vi "Circus FPGA List.vi"(6 "Init":bool, 8 "error in (no error)":errorcluster) -> (0 "error out":errorcluster, 3 "FPGA List out":string[](array[string]))   [LabVIEW 2026, in "TALOS.lvlib"]
doc: "This VI contains the list of all the AEgIS PCs names (machine names)."
uses:
  TALOS.lvlib
  Global Memory.vi
  Interfaces/FPGA Interface/FPGA Interface.lvclass
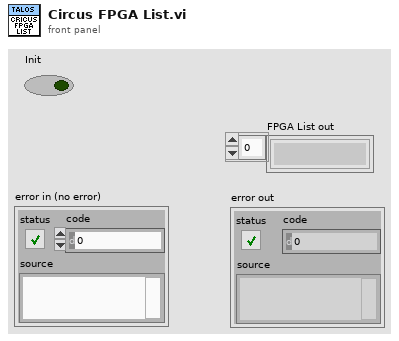
[diagram p1: front panel]
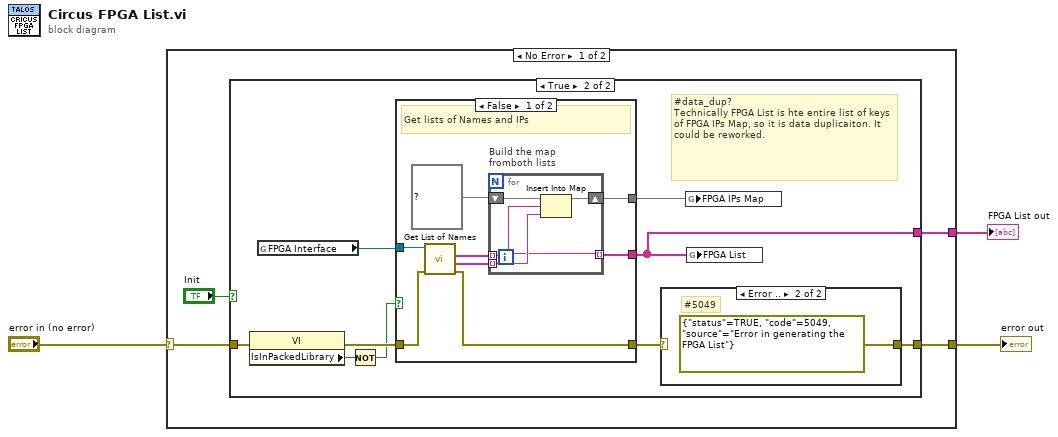
[diagram p0: block diagram]
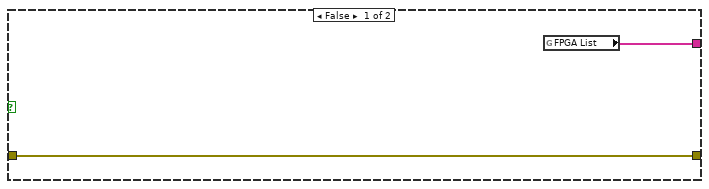
[diagram p2: hidden frame]
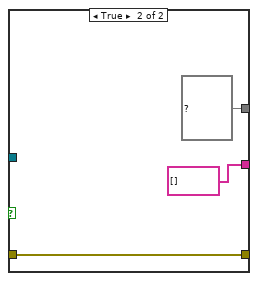
[diagram p3: hidden frame]
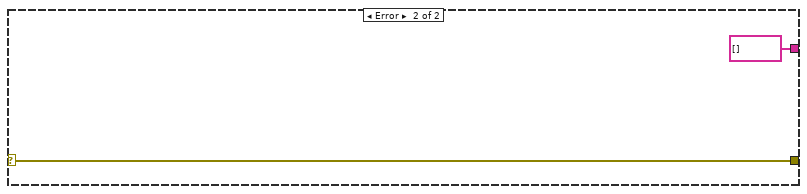
[diagram p5: hidden frame]
diagram:
  n1 = case shown="No Error" "error in (no error)" {
    selector: "error in (no error)" -> [w6 w36]
    tunnel: [w7 w36] -> w3
    tunnel: [w5 string[] [] ("FPGA List")] -> w1
    frame No Error {
      n2 = case shown="True" "Init" {
        tunnel: [w8 w15] -> w5
        tunnel: w6 -> [w9 w18]
        tunnel: [w9 w13] -> w7
        frame False {
          n3 = global read "Global Memory.vi" "FPGA List"() -> (w8:string[])
        }
        frame True {
          # "#data_dup?\nTechnically FPGA List is hte entire list of keys of FPGA IPs Map, so it is data duplicaiton. It could be reworked."
          n4 = property class="VI"(error in=w18) -> (error out=w17:errorcluster, "IsInPackedLibrary"=w16:bool)  [unwired: 1 in, 1 out]
          n5 = global read "Global Memory.vi" "FPGA Interface"() -> (w10:refnum<class "FPGA Interface.lvclass">)
          n6 = Not(x=w16) -> (.not. x?=w12:bool)
          n7 = case shown="False" w12 {
            tunnel: [w19 string[] []] -> w15
            tunnel: w17 -> [w24 w33]
            tunnel: [w25 w33] -> w14
            tunnel: w10 -> [w26 _]
            tunnel: [w22 map{string, string} {} ("FPGA IPs Map")] -> w11
            frame False {
              # "Get lists of Names and IPs"
              n8 = call-dynamic "Get List of Names.vi"("error in (no error)"=w24, "FPGA Interface in"=w26) -> ("error out"=w25:errorcluster, "List of IPs"=w20:string[], "List of Names"=w21:string[])  [unwired: 6 in, 1 out]
              n9 = for "Build the map\nfromboth lists" {
                shift-right: [w29] -> w22
                shift-left: map{string, string} {} ("FPGA IPs Map") -> [w30]
                tunnel: w21 -> [w27] mode=indexing
                tunnel: w20 -> [w28] mode=indexing
                tunnel: [w27] -> w19 mode=indexing
                n10 = Insert Into Map(map in=w30, key=w27, value=w28) -> (map out=w29:map{string, string})  [unwired: 2 out]
              }
            }
            frame True {
            }
          }
          n11 = case shown="Error .." w14 {
            selector: w14 -> [w34 _]
            tunnel: [w34 errorcluster {"status"=TRUE, "code"=5049, "source"="Error in generating the FPGA List"} ("error IO")] -> w13
            frame No Error {
            }
            frame Error {
              # "#5049"
            }
          }
          n12 = global write "Global Memory.vi" "FPGA IPs Map"(w11) -> ()
          n13 = global write "Global Memory.vi" "FPGA List"(w15) -> ()
        }
      }
    }
    frame Error {
    }
  }
  "FPGA List out" <- w1
  "error out" <- w3
